vi "TharOpen.vi"(8 "error in (no error)":errorcluster, 11 "Device Serial Number":string) -> (0 "error constant":errorcluster, 3 "Handle":u32)   [LabVIEW 2016]
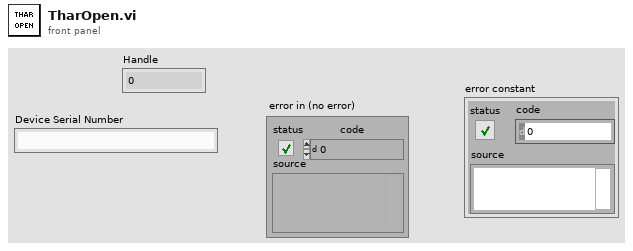
[diagram p1: front panel]
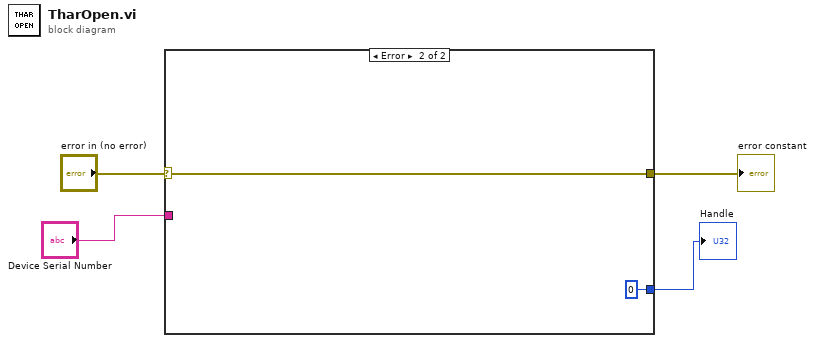
[diagram p0: block diagram]
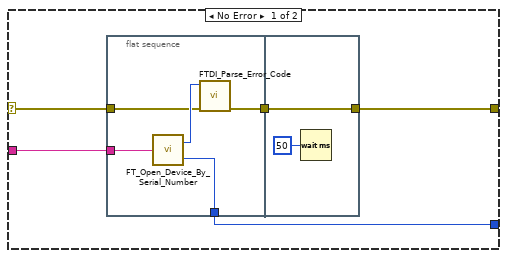
[diagram p2: hidden frame]
diagram:
  n1 = case shown="Error" "error in (no error)" {
    selector: "error in (no error)" -> [w8 w18]
    tunnel: [w9 w18] -> w4
    tunnel: "Device Serial Number" -> [w7 _]
    tunnel: [w5 u32 0 ("Handle")] -> w1
    frame No Error {
      n2 = flat-sequence {
        tunnel: w8 -> [w12]
        tunnel: w7 -> [w11]
        tunnel: [w13] -> w6
        tunnel: [w10] -> w5
        tunnel: [w16] -> w9
        tunnel: w6 -> [w16]
        frame #0 {
          n3 = call "FT_Open_Device_By_Serial_Number.vi"("Device Serial Number"=w11) -> ("FT_Status"=w14:u32, "Handle"=w10:u32)
          n4 = call "FTDI_Parse_Error_Code.vi"("error in (no error)"=w12, "FT_Status"=w14) -> ("error out"=w13:errorcluster)  [unwired: 9 in]
        }
        frame #1 {
          n5 = Wait (ms)(milliseconds to wait=u32 50) -> ()  [unwired: 1 out]
        }
      }
    }
    frame Error {
    }
  }
  "error constant" <- w4
  "Handle" <- w1
